vi "Write Value.vi"(8 "error in (no error)":errorcluster, 10 "Data":T1=variant(timestamp timestamp(0 s since 1904-01-01)), 11 "Numeric in":refnum<class "Const_Variant.lvclass">) -> (0 "error out":errorcluster, 3 "Numeric out":refnum<class "Const_Variant.lvclass">)   [LabVIEW 2021, in "Const_Variant.lvclass"]
uses:
  Const_Variant.lvclass
  Type.ctl
  Const_Variant.lvclass/Const_Variant.ctl
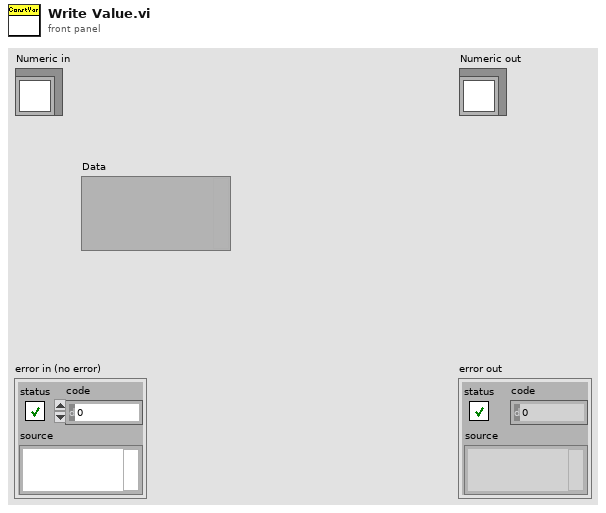
[diagram p1: front panel]
types:
  T1 = typedef "Const_Variant.lvclass/Type.ctl" = variant
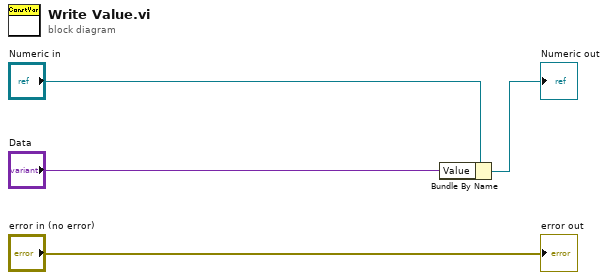
[diagram p0: block diagram]
diagram:
  n1 = Bundle By Name(cluster="Numeric in", "Value"="Data") -> (→"Numeric out":refnum<class "Const_Variant.lvclass">)
  "error out" <- "error in (no error)"
